vi "Scope_5782_6channel.vi"() -> ()   [LabVIEW 2018]
uses:
  FPGA/DataMode.ctl
  <vilib>/Analysis/4window.llb/windowTd.ctl
  Host/Scope/controls/power_spectrum_unit.ctl
  Host/Scope5782/Scope/controls/5782_trigger_type.ctl
  Host/Scope/controls/Data_calc_mode.ctl
  Host/Scope/controls/Data_display_mode.ctl
  Host/Scope/controls/Graph_references.ctl
  Host/Scope/controls/graph_controls.ctl
  Host/Scope/controls/Channel_select_2fpga.ctl
  <vilib>/userdefined/High Color/nirio_resource_hc.ctl
  Host/Communication/Driver/RemoteConnection/RemoteReferences.ctl
  Host/FpgaRef/FpgaRef5761/ClockSource_5761.ctl
  Host/Scope/Scope5782_six_channel/Scope5782_six_channel.lvclass
  C:/PXIe/Workspace/Host/Scope/ScopeBase/ScopeBase.lvclass
  Host/Communication/Driver/RemoteConnection/RemoteConnection.lvclass
  Host/Scope/ScopeBase/ScopeBase.lvclass/ScopeBase.ctl
  FPGA/fpga_settings.ctl
  Host/Scope/Scope5782_six_channel/Scope5782_six_channel.lvclass/Scope5782_six_channel.ctl
  Host/Scope/controls/ScopeMode.ctl
  Host/FpgaRef/FpgaRef5761/FpgaRef5761.lvclass
  C:/PXIe/Workspace/Host/FpgaRef/FpgaRefBase/FpgaRefBase.lvclass
  Host/FpgaRef/FpgaRef5782/FpgaRef5782.lvclass
  Host/Communication/global_stop.vi
  <vilib>/FPGAPlugInAG/PXIe-7975R/niLvFpga_Open_PXIe-7975R.vi
  <vilib>/rvi/interface/common/dynamic/niFpgaDynamicAddResources.vi
  Host/Communication/response.ctl
  Host/Communication/driver_status.ctl
  <vilib>/rvi/interface/nirviOpenFPGA/nirviOpenFPGA.xnode
  FPGA Bitfiles/FPGAmain_5782_Fast_PID_X3R1Zvw8vDM.lvbitx
  FPGA Bitfiles/FPGAmain_5761_zuew0qNtRjU.lvbitx
  <vilib>/rvi/FXPMathLib/FxpInterpret/XNode/nifxpmath_Interpret.xnode
  Host/Communication/Driver/TcpServerDriver/TcpServerDriver.lvclass
  Host/Scope/ScopeBase/ScopeBase.lvclass
  Host/FpgaRef/FpgaRefBase/FpgaRefBase.lvclass
  <vilib>/Analysis/NI_AALPro.lvlib
panel:
  in  "Tab Control":T1(tab)
  in  "Fequency [kHz]":dbl format="%#_8g"
  in  "a":fxp<+/-,16,2>
  in  "b":fxp<+/-,16,2>
  in  "Feedback":bool
  in  "Ki*T":fxp<+/-,32,4>
  in  "Kd/T":fxp<+/-,32,4>
  in  "Kp":fxp<+/-,32,4>
  in  "Feedback AM":bool caption="Feedback"
  in  "Ki*T AM":fxp<+/-,32,4> caption="Ki*T"
  in  "Kd/T AM":fxp<+/-,32,4> caption="Kd/T"
  in  "Kp AM":fxp<+/-,32,4> caption="Kp"
  in  "Feedback delay":u32
  in  "Trigger delay":u32
  in  "Acquire samples":u32
  in  "ch2 DC offset":dbl caption="DC offset\nChannel 2"
  in  "ch3 DC offset":dbl caption="DC offset\nChannel 3"
  in  "ch0 DC offset 2":dbl caption="DC offset\nChannel 0"
  in  "ch1 DC offset 2":dbl caption="DC offset\nChannel 1"
  in  "ch0 DC offset":dbl caption="DC offset\nChannel 0"
  in  "ch1 DC offset":dbl caption="DC offset\nChannel 1"
  in  "Setpoint":path
  in  "Beam":path
  in  "Feed forward":path
  in  "show setpoint":bool
  in  "show beam":bool
  in  "show feedforward":bool
  in  "Setpoint enabled":bool
  in  "Beam/FF enabled":bool
  in  "Cavity model":bool
  in  "w12":dbl format="%#_12g"
  in  "R1":dbl
  in  "w1":dbl
  in  "Q1":dbl
  in  "K1":dbl
  in  "S":dbl=0.001 min=0.001 max=1000.0 format="%#_12g"
  in  "Input delay 5761":u32
  in  "Input delay 5782":u32
  in  "5761 resource":T2="PXI2Slot11"
  in  "5782 resource":T2="PXI2Slot18"
  in  "High speed transfer to host":bool=TRUE
  in  "Output enabled":bool=TRUE
  in  "Output delay delta":dbl(slide) scale=0.0..6.0
  in  "Output delay":dbl(slide) scale=0.0..6.0
  in  "Output mixer fequency [MHz]":dbl
  in  "Trigger":T3
  in  "Mode":T4
  in  "Mixer freq [MHz]":dbl
  in  "unwrap phase":bool
  in  "#bins":i32=1 min=1 max=16
  in  "Unit":T5
  in  "Window":T6=1 items=["Rectangle"=0, "Hanning"=1, "Hamming"=2, "Blackman-Harris"=3, "Exact Blackman"=4, "Blackman"=5, "Flat Top"=6, "4 Term B-Harris "=7, "7 Term B-Harris"=8, "Low Sidelobe"=9, "Blackman Nuttall"=11, "Triangle"=30, "Bartlett-Hanning"=31, "Bohman"=32, "Parzen"=33, "Welch"=34, "Kaiser"=60, "Dolph-Chebyshev"=61, "Gaussian"=62]
  in  "Chart length":i32=400000
  in  "Trigmode":enum32{"Triggered", "Continuous"}(radio)
  in  "Reference for phase":T7
  in  "Graph_refs":T8
  out "Lower chart":dbl[][](graph)
  out "Upper chart":dbl[][](graph)
  out "Lower graph":i16[][](graph)
  in  "Buffer":T10
  in  "Display":T11
  out "stop 2":bool
  in  "Zoom freq X":bool
  in  "Zoom freq Y":bool
  in  "Zoom time Y":bool
  in  "Zoom time X":bool
  in  "Samples per 5782 record":i32
  in  "Phase offset (deg)":dbl
  in  "Fequency [MHz]":dbl format="%#_8g"
  out "freqdata":cluster{"f0":dbl, "df":dbl, "magnitude":dbl[]}[](graph)
  out "Upper graph":i16[][](graph)
  in  "Rumode":bool
  in  "Singleshot":bool
  out "error IO":errorcluster
  in  "stop":bool
  # "FPGA setup"
  # "ns"
  # "Output delay"
  # "ps"
  # "Output delay delta"
  # "Auto Zoom"
  # "FFT"
  # "Auto Zoom"
  # "Amplitude modulation"
  # "Phase"
  # "Amplitude"
  # "Delays"
  # "5782"
  # "V"
  # "V"
  # "5761"
  # "V"
  # "V"
  # "V"
  # "V"
  # "Simulated data"
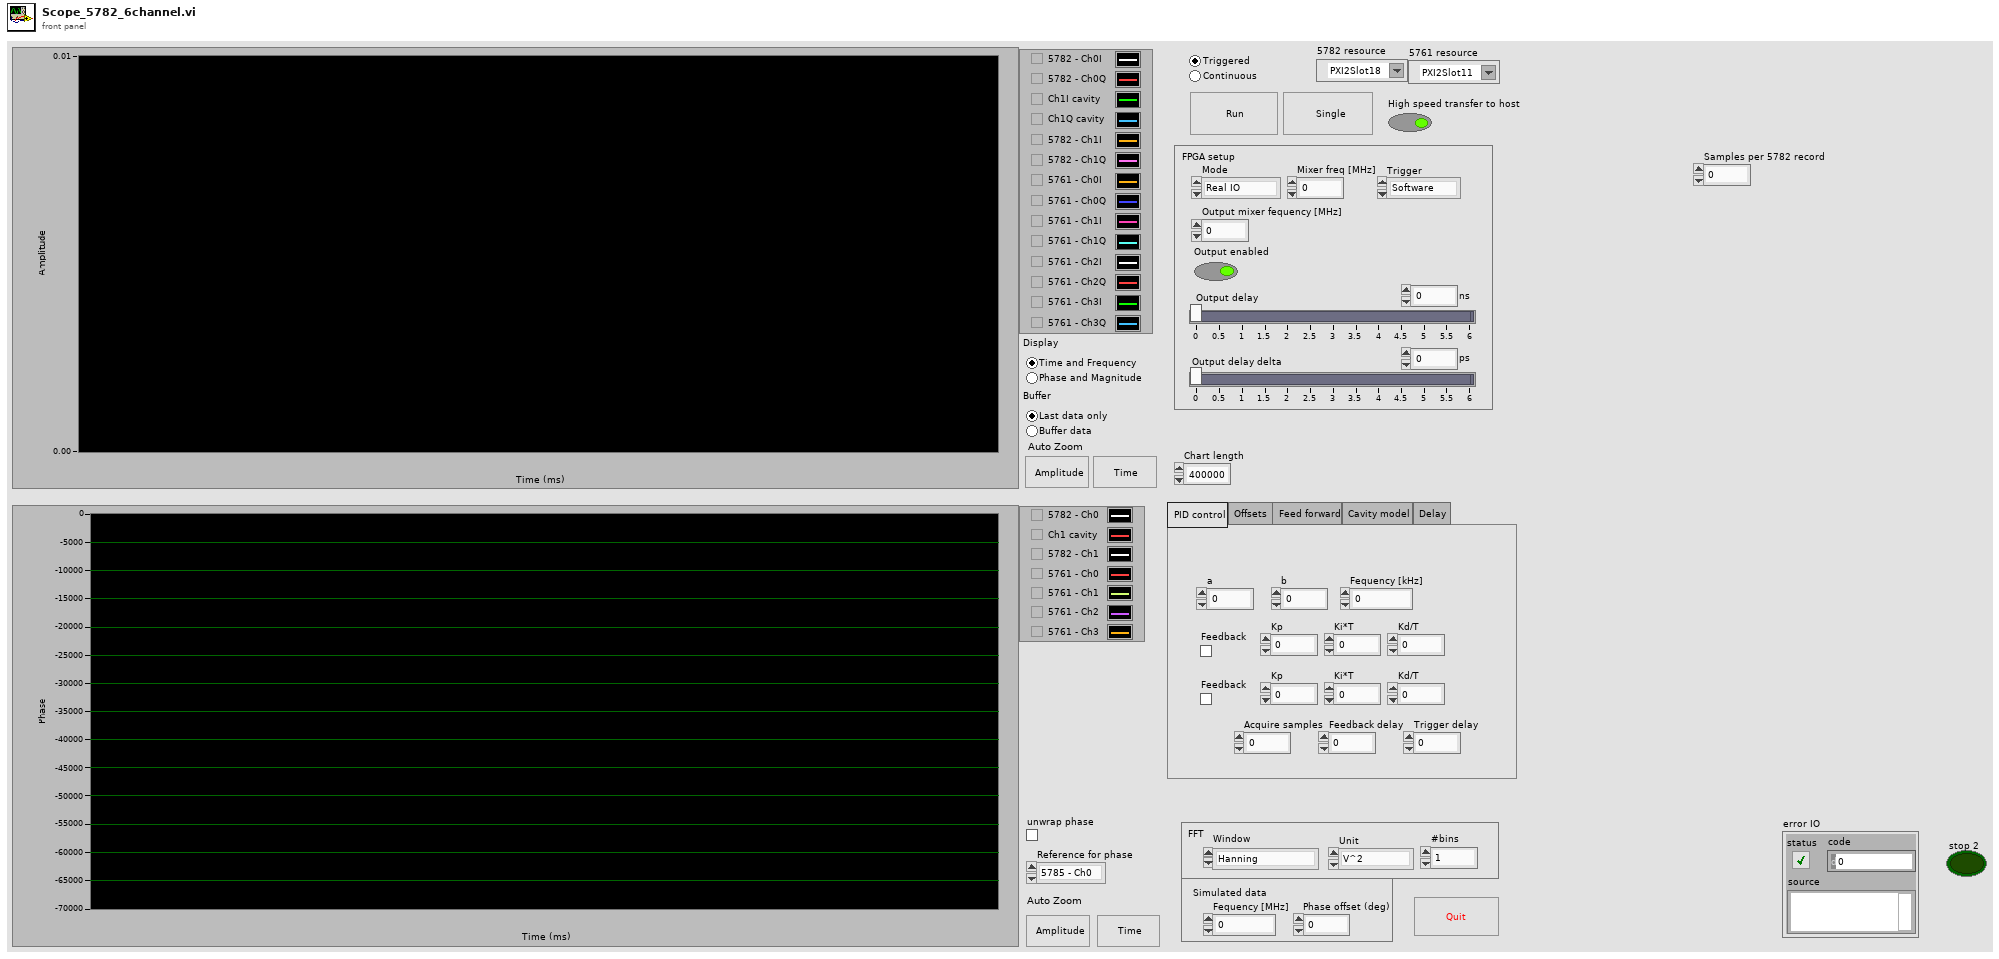
[diagram p1: front panel]
types:
  T1 = enum32{"PID control", "Offsets", "Feed forward", "Cavity model", "Delay"}
  T2 = typedef "nirio_resource_hc.ctl" = tag
  T3 = typedef "5782_trigger_type.ctl" = enum16{"Software", "Trigger input"}
  T4 = typedef "DataMode.ctl" = enum16{"Real IO", "Simulated"}
  T5 = typedef "power_spectrum_unit.ctl" = enum16{"V^2", "V", "dBV"}
  T6 = typedef "NI_AALPro.lvlib/windowTd.ctl" = u32
  T7 = typedef "Channel_select_2fpga.ctl" = enum16{"5785 - Ch0", "5785 - Ch1 cavity", "5785 - Ch1", "5761 - Ch0", "5761 - Ch1", "5761 - Ch2", "5761 - Ch3"}
  T8 = typedef "Graph_references.ctl" = cluster{"upper":T9, "lower":T9, "Freq graph":refnum<vi>}
  T9 = typedef "graph_controls.ctl" = cluster{"Graph":refnum<vi>, "Time btn":refnum<vi>, "Amplitude btn":refnum<vi>, "Chart":refnum<vi>}
  T10 = typedef "Data_display_mode.ctl" = enum32{"Last data only", "Buffer data"}
  T11 = typedef "Data_calc_mode.ctl" = enum32{"Time and Frequency", "Phase and Magnitude"}
  T12 = enum8{"Internal Clock PLL Off", "Internal Clock PLL On (REF IN)", "External Clock (CLK_IN)", "Internal Clock PLL On (IoModSyncClk)"}
  T13 = typedef "ClockSource_5761.ctl" = enum8{"Internal Clock PLL Off", "Internal Clock PLL On (CLK_IN)", "External Clock (CLK_IN)", "Internal Clock PLL On (IoModSyncClk)", "External Clock (IoModSyncClk)"}
  T14 = typedef "RemoteConnection.lvclass/RemoteReferences.ctl" = cluster{"a":refnum<vi>, "b":refnum<vi>, "fm":refnum<vi>, "Output delay":refnum<vi>, "Output delay delta":refnum<vi>}
  T15 = typedef "response.ctl" = cluster{"driver status":T16, "Sender":string, "Type":i32, "Variant":variant}
  T16 = typedef "driver_status.ctl" = enum16{"Normal", "Startup", "Connection lost", "Reconnected", "Timeout", "Idle", "Busy"}
  T17 = typedef "message_queue.ctl" = refnum<queue>
  T18 = typedef "fpga_settings.ctl" = enum16{"Feedback Enable", "New FIR coeffs", "FIR shift", "Enable filter", "Set Downsample", "Downsample", "CIC Gain", "Record length", "Trigger samples", "Quiet time", "a_am", "b_am", "Use fixed delay", "fixed sin_fi", "fixed cos_fi", "Ki*Tau", "Kp", "Kd_Tau", "Fi_start", "Fi_delta", "DC_offs 0", "DC_offs 1", "DC_offs 2", "DC_offs 3", "Ki*Tau am", "Kp am", "Kd_Tau am", "Feedback AM", "Trigger delay", "Feedback delay", "Setpoint enable", "Beam enable", "Samples to acquire", "Cavity Enable", "Cavity C1", "Cavity C2", "Cavity C3", "Cavity C4", "Cavity C5", "Input delay"}
  T19 = typedef "ScopeMode.ctl" = enum16{"Stopped", "Single", "Running", "Continuous"}
  T20 = typedef "Feedforward.ctl" = cluster{"Beam I":dbl[], "Beam Q":dbl[], "Feedforward I":dbl[], "Feedforward Q":dbl[], "Setpoint I":dbl[], "Setpoint Q":dbl[]}
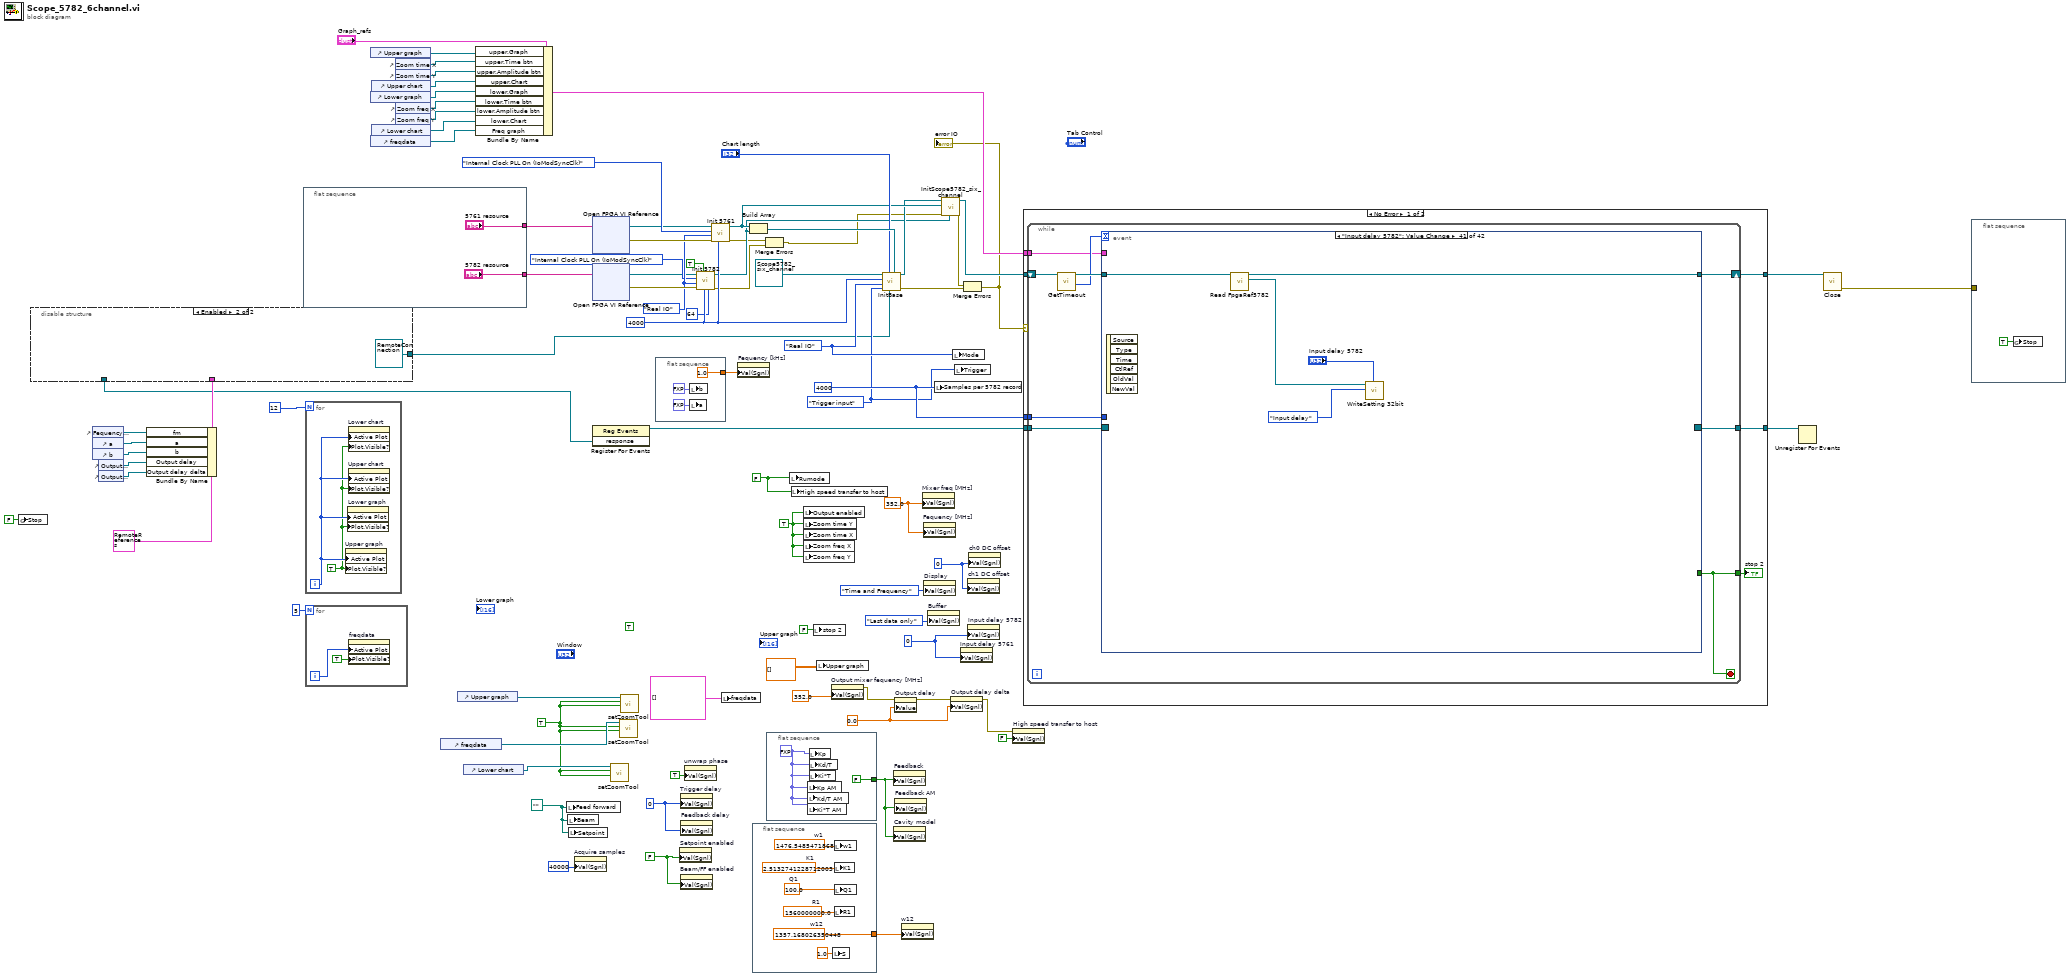
[diagram p0: block diagram]
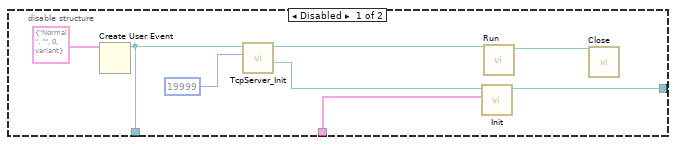
[diagram p2: hidden frame]
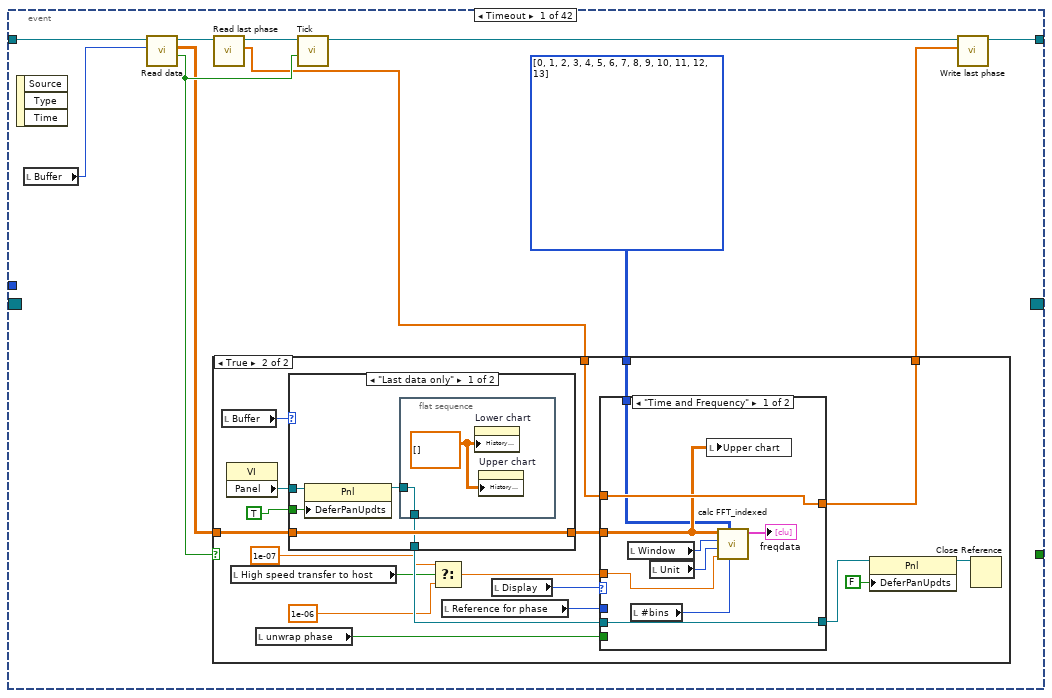
[diagram p3: hidden frame]
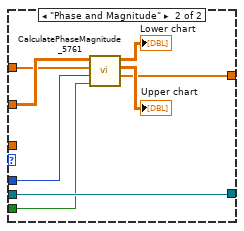
[diagram p6: hidden frame]
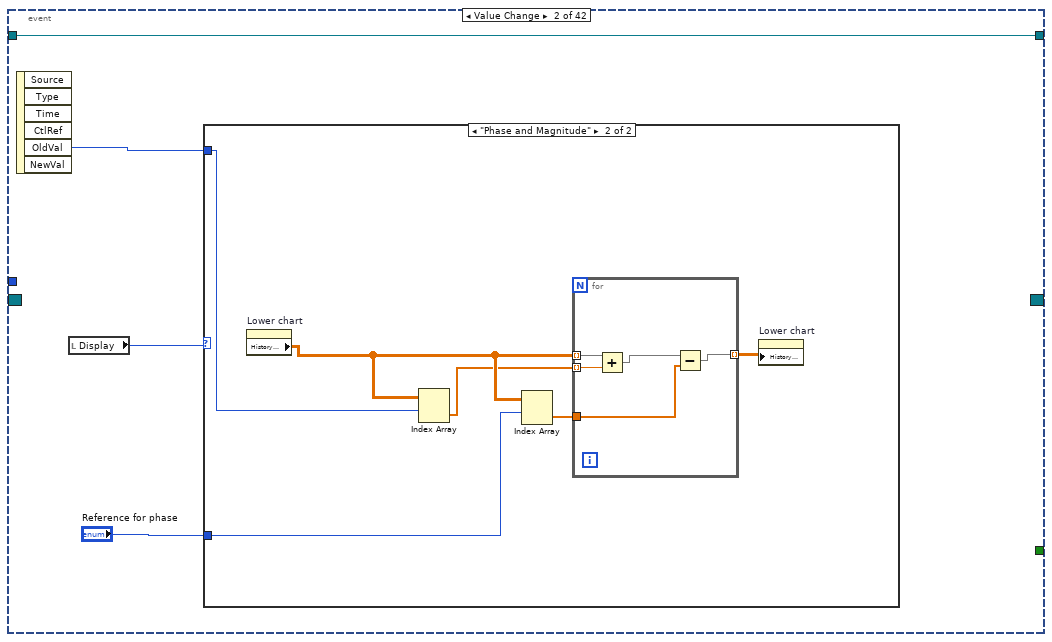
[diagram p7: hidden frame]
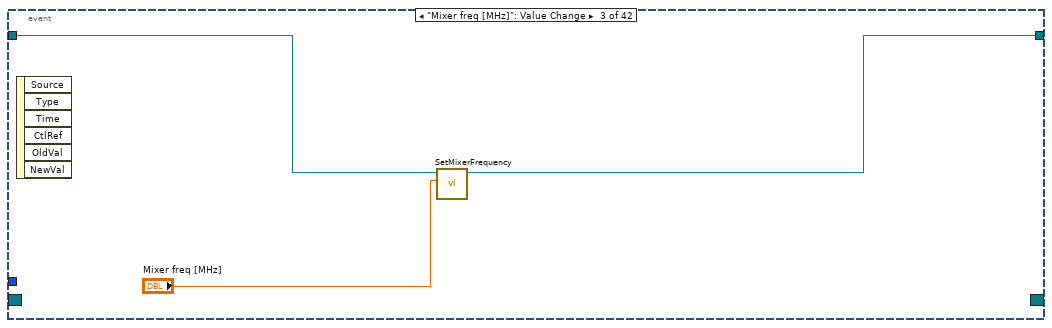
[diagram p9: hidden frame]
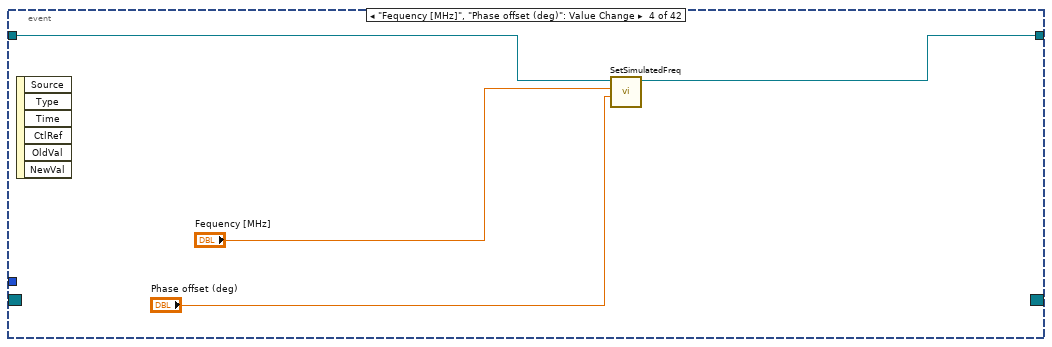
[diagram p10: hidden frame]
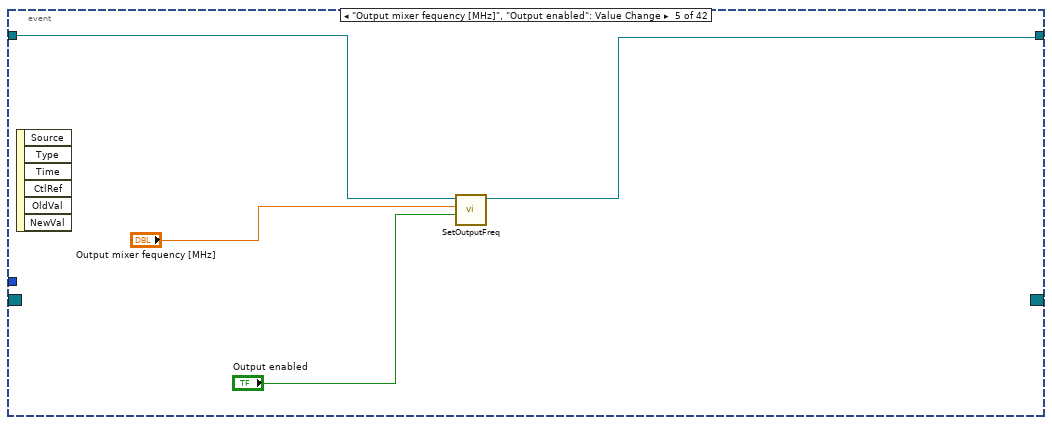
[diagram p11: hidden frame]
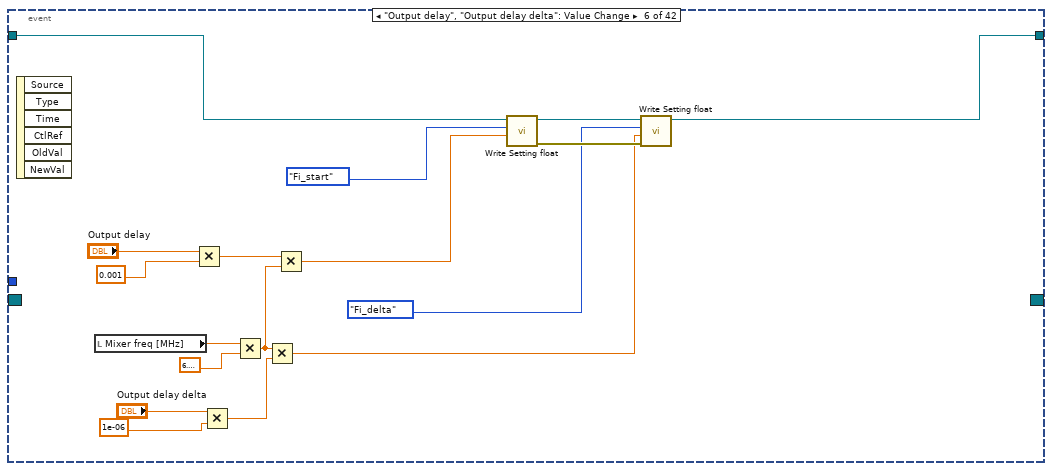
[diagram p12: hidden frame]
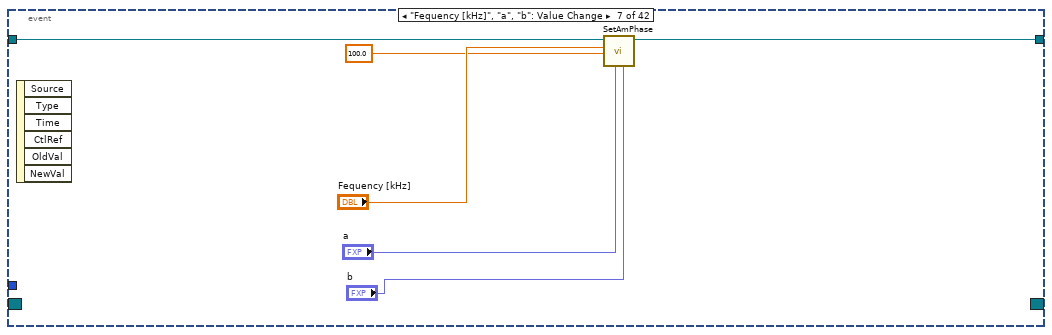
[diagram p13: hidden frame]
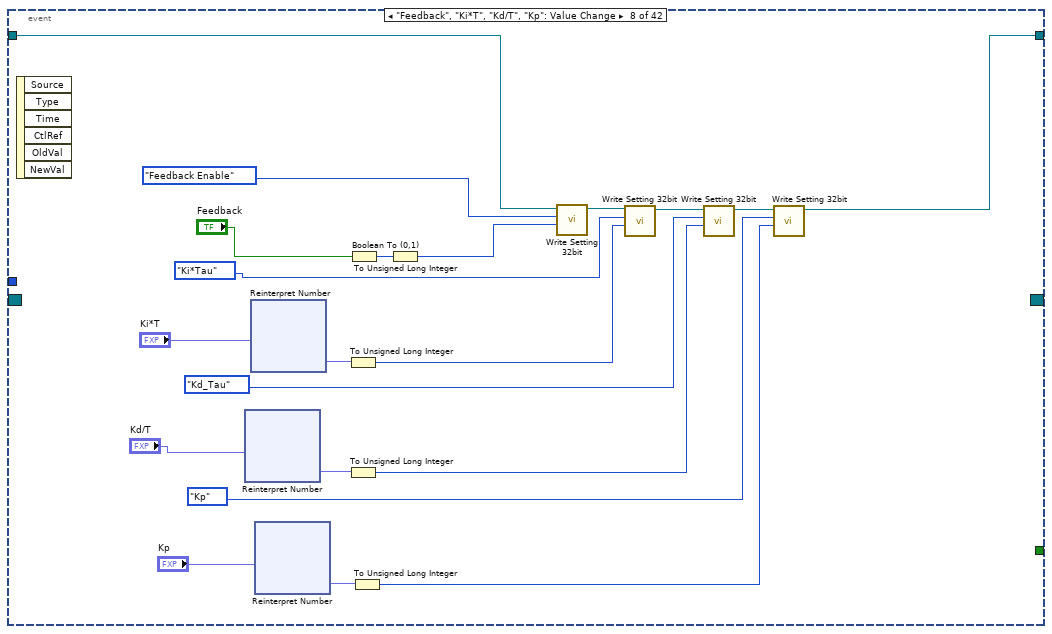
[diagram p14: hidden frame]
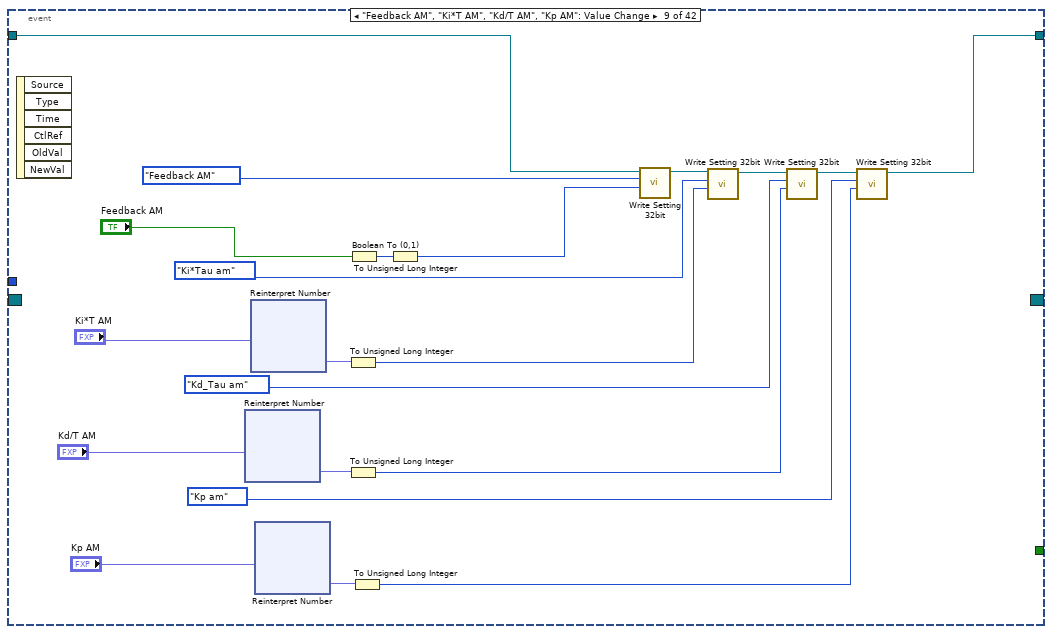
[diagram p15: hidden frame]
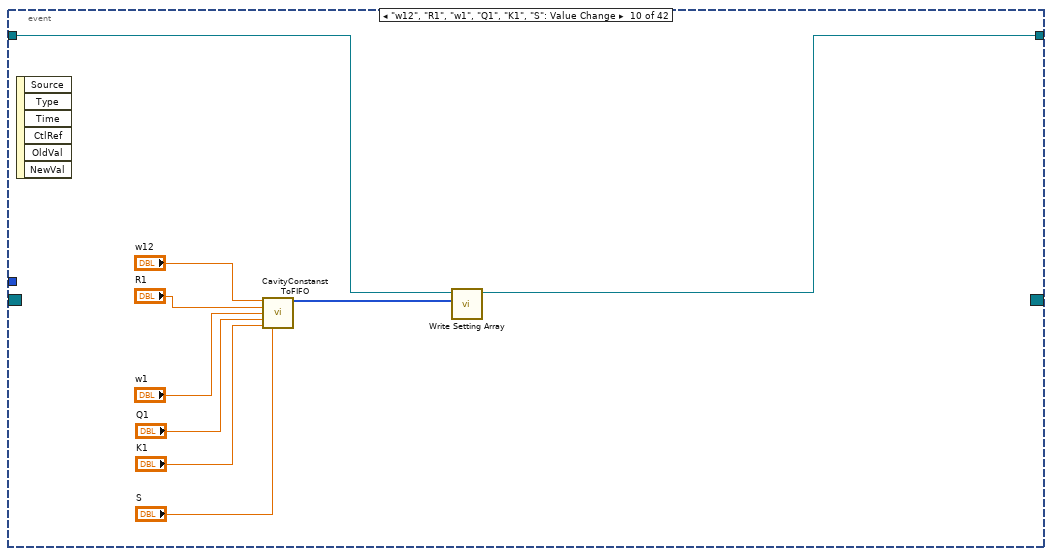
[diagram p16: hidden frame]
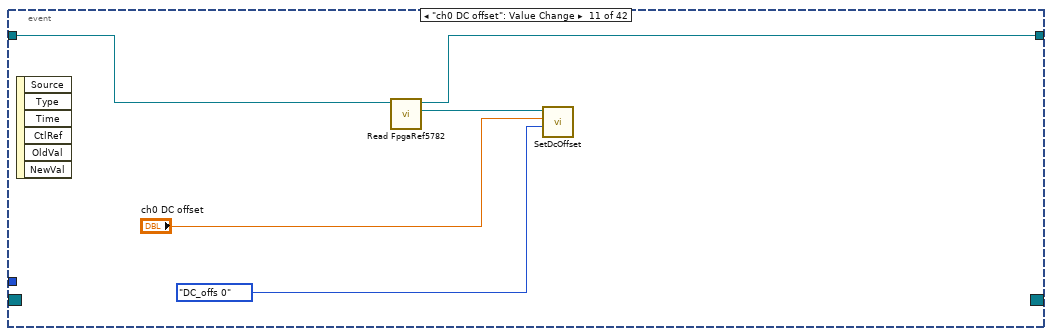
[diagram p17: hidden frame]
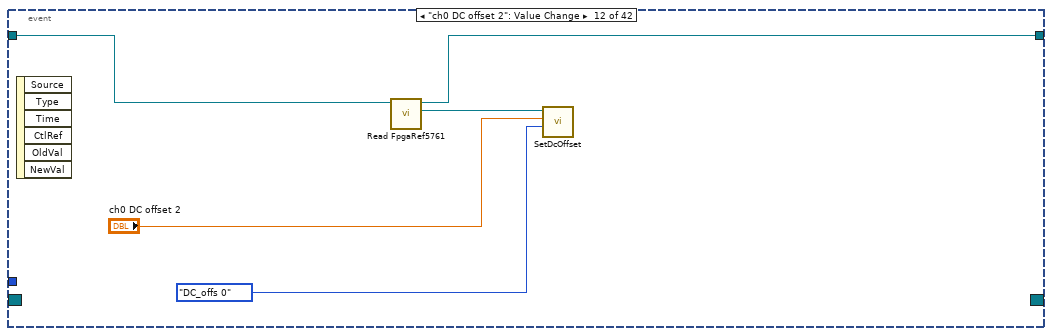
[diagram p18: hidden frame]
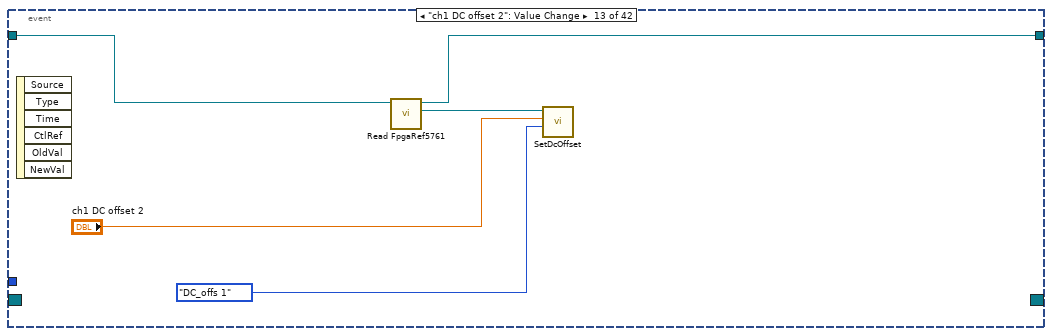
[diagram p19: hidden frame]
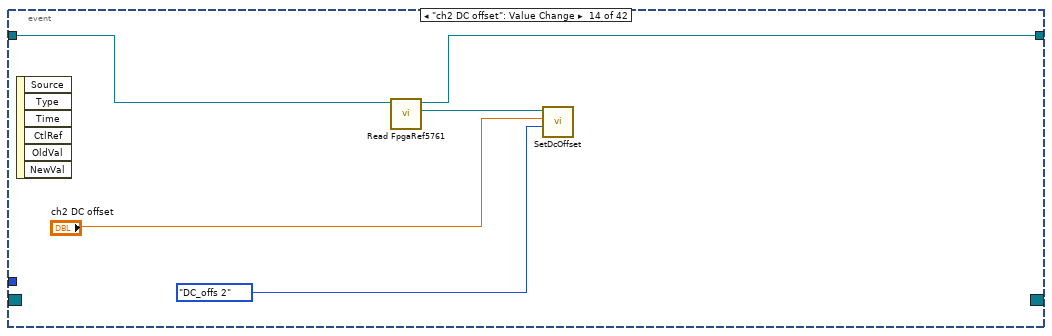
[diagram p20: hidden frame]
diagram:
  w1 = u32 0 ("Value (Signaling)")
  w18 = u16 4000 ("Samples to aqcuire")
  w14 = DataMode."Real IO" ("Mode")
  w27 = DataMode."Real IO" ("Mode")
  w35 = path "" ("Feed forward")
  w36 = FALSE ("Value (Signaling)")
  w37 = u32 0 ("Value (Signaling)")
  w56 = i16 0 ("Value (Signaling)")
  w57 = 0.0 ("Value (Signaling)")
  w26 = 5782_trigger_type."Trigger input" ("Trigger")
  w46 = TRUE ("Zoom  X")
  w42 = TRUE ("Rumode")
  w41 = 4000 ("Samples to aqcuire")
  (unwired) TRUE ("Rumode")
  w40 = FALSE ("Rumode")
  w81 = 352.0 ("Mixer requency [MHz]")
  n1 = global write "global_stop.vi" "Stop"(FALSE ("Stop")) -> ()
  n2 = control-ref of="Fequency [kHz]"() -> (w50:refnum<vi>)
  n3 = control-ref of="a"() -> (w51:refnum<vi>)
  n4 = control-ref of="b"() -> (w49:refnum<vi>)
  n5 = control-ref of="Output delay"() -> (w45:refnum<vi>)
  n6 = control-ref of="Output delay delta"() -> (w44:refnum<vi>)
  n7 = Bundle By Name(cluster=T14 {"a"=refnum, "b"=refnum, "fm"=refnum, "Output delay"=refnum, "Output delay delta"=refnum} ("refs"), "fm"=w50, "a"=w51, "b"=w49, "Output delay"=w45, "Output delay delta"=w44) -> (w54:T14)
  n8 = disable-structure shown="Enabled" {
    disable-tunnel: w54 -> [w91 _]
    disable-tunnel: [w86 _] -> w48
    disable-tunnel: [w84 refnum<class "RemoteConnection.lvclass"> refnum ("RemoteConnection")] -> w25
    frame Disabled {
      n9 = Create User Event(user event datatype=T15 {"driver status"=enum."Normal", "Sender"="", "Type"=0, "Variant"=variant} ("response")) -> (user event=w86:refnum<user-event>)  [unwired: 1 in, 1 out]
      n10 = call "TcpServer_Init.vi"("local port"=u16 19999, "response event"=w86) -> ("Message queue"=w90:T17, "TcpServerDriver"=w88:refnum<class "TcpServerDriver.lvclass">)  [unwired: 8 in]
      n11 = call "Init.vi"("refs"=w91, "server queue"=w90) -> ("RemoteConnection"=w84:refnum<class "RemoteConnection.lvclass">)  [unwired: 9 in]
      n12 = call-dynamic "Run.vi"("BaseDriver in"=w88) -> ("BaseDriver out"=w89:refnum<class "TcpServerDriver.lvclass">)  [unwired: 9 in, 1 out]
      n13 = call-dynamic "Close.vi"("BaseDriver in"=w89) -> ()  [unwired: 9 in, 2 out]
    }
    frame Enabled {
    }
  }
  n14 = flat-sequence {
    tunnel: ["5761 resource"] -> w29
    tunnel: ["5782 resource"] -> w28
    frame #0 {
    }
  }
  n15 = for {
    N: 12 -> [_]
    i -> [w96]
    w95 = TRUE ("Plot.Visible")
    n16 = property on="Upper graph" class="WFGraph (strict)"("Active Plot"=w96, "Plot.Visible?"=w95) -> ()  [unwired: 2 in, 2 out]
    n17 = property on="Lower graph" class="WFGraph (strict)"("Active Plot"=w96, "Plot.Visible?"=w95) -> ()  [unwired: 2 in, 2 out]
    n18 = property on="Lower chart" class="WFChart (strict)"("Active Plot"=w96, "Plot.Visible?"=w95) -> ()  [unwired: 2 in, 2 out]
    n19 = property on="Upper chart" class="WFChart (strict)"("Active Plot"=w96, "Plot.Visible?"=w95) -> ()  [unwired: 2 in, 2 out]
  }
  n20 = for {
    N: 5 -> [_]
    i -> [w97]
    n21 = property on="freqdata" class="WFGraph (strict)"("Active Plot"=w97, "Plot.Visible?"=TRUE ("Plot.Visible")) -> ()  [unwired: 2 in, 2 out]
  }
  n22 = control-ref of="Upper graph"() -> (w71:refnum<vi>)
  n23 = control-ref of="Lower graph"() -> (w67:refnum<vi>)
  n24 = control-ref of="freqdata"() -> (w63:refnum<vi>)
  n25 = control-ref of="Upper chart"() -> (w68:refnum<vi>)
  n26 = control-ref of="Lower chart"() -> (w64:refnum<vi>)
  n27 = control-ref of="Zoom time X"() -> (w70:refnum<vi>)
  n28 = control-ref of="Zoom time Y"() -> (w69:refnum<vi>)
  n29 = control-ref of="Zoom freq X"() -> (w66:refnum<vi>)
  n30 = control-ref of="Zoom freq Y"() -> (w65:refnum<vi>)
  n31 = control-ref of="freqdata"() -> (w74:refnum<vi>)
  n32 = control-ref of="Upper graph"() -> (w75:refnum<vi>)
  n33 = control-ref of="Lower chart"() -> (w47:refnum<vi>)
  n34 = Bundle By Name(cluster="Graph_refs", "upper.Graph"=w71, "upper.Time btn"=w70, "upper.Amplitude btn"=w69, "upper.Chart"=w68, "lower.Graph"=w67, "lower.Time btn"=w66, "lower.Amplitude btn"=w65, "lower.Chart"=w64, "Freq graph"=w63) -> (w62:T8)
  n35 = local write "Feed forward"(w35) -> ()
  n36 = local write "Beam"(w35) -> ()
  n37 = local write "Setpoint"(w35) -> ()
  n38 = property on="Acquire samples" class="DigNum (strict)"("Val(Sgnl)"=u32 40000 ("Value (Signaling)")) -> ()  [unwired: 2 in, 2 out]
  n39 = register-events(w48) -> (reference out=w78:refnum<event-registration>)  [unwired: 2 in, 1 out]
  n40 = xnode "Open FPGA VI Reference"("resource name"=w29) -> ("FPGA VI Reference Out"=w2:refnum<k20>, "error out"=w16:errorcluster)  [unwired: 1 in]
  n41 = xnode "Open FPGA VI Reference"("resource name"=w28) -> ("FPGA VI Reference Out"=w3:refnum<k20>, "error out"=w17:errorcluster)  [unwired: 1 in]
  n42 = call "setZoomTool.vi"("Zoom Y"=w46, "Zoom  X"=w46, "reference"=w47) -> ()  [unwired: 9 in]
  n43 = call "setZoomTool.vi"("Zoom Y"=w46, "Zoom  X"=w46, "reference"=w74) -> ()  [unwired: 9 in]
  n44 = call "setZoomTool.vi"("Zoom Y"=w46, "Zoom  X"=w46, "reference"=w75) -> ()  [unwired: 9 in]
  n45 = flat-sequence {
    tunnel: [1.0 ("Value (Signaling)")] -> w55
    frame #0 {
      n46 = local write "b"(fxp<+/-,16,2> 0.0 ("b")) -> ()
      n47 = local write "a"(fxp<+/-,16,2> 1.0 ("a")) -> ()
    }
  }
  n48 = property on="Setpoint enabled" class="Bool (strict)"("Val(Sgnl)"=w36) -> ()  [unwired: 2 in, 2 out]
  n49 = property on="Trigger delay" class="DigNum (strict)"("Val(Sgnl)"=w37) -> ()  [unwired: 2 in, 2 out]
  n50 = property on="Beam/FF enabled" class="Bool (strict)"("Val(Sgnl)"=w36) -> ()  [unwired: 2 in, 2 out]
  n51 = property on="Feedback delay" class="DigNum (strict)"("Val(Sgnl)"=w37) -> ()  [unwired: 2 in, 2 out]
  n52 = property on="unwrap phase" class="Bool (strict)"("Val(Sgnl)"=TRUE ("Value (Signaling)")) -> ()  [unwired: 2 in, 2 out]
  n53 = call "Init 5782.vi"("User Data 1"=u8 64, "Record length"=w18, "Use 1Mhz clock"=TRUE, "error in (no error)"=w17, "Mode"=w14, "Clock Source"=T12."Internal Clock PLL On (IoModSyncClk)", "FPGA ref"=w3) -> ("error out"=w8:errorcluster, "FpgaRef5782 Out"=w11:refnum<class "FpgaRef5782.lvclass">)  [unwired: 3 in]
  n54 = call "Init 5761.vi"("Record length"=w18, "error in (no error)"=w16, "Mode"=w14, "Clock Source"=ClockSource_5761."Internal Clock PLL On (IoModSyncClk)", "FPGA ref"=w2) -> ("error out"=w9:errorcluster, "FpgaRef5761 out"=w21:refnum<class "FpgaRef5761.lvclass">)  [unwired: 5 in]
  n55 = local write "freqdata"(cluster{"f0":dbl, "df":dbl, "magnitude":dbl[]}[] [] ("freqdata")) -> ()
  n56 = property on="Fequency [kHz]" class="DigNum (strict)"("Val(Sgnl)"=w55) -> ()  [unwired: 2 in, 2 out]
  n57 = Build Array(w21, w11) -> (w30:refnum<class "FpgaRefBase.lvclass">[])
  n58 = flat-sequence {
    tunnel: [w103] -> w32
    frame #0 {
      w104 = 2.5132741228712003  # K1
      w105 = 100.0  # Q1
      w106 = 1476.54854718683  # w1
      w107 = 1560000000.0  # R1
      w103 = 1357.168026350448  # w12
      n59 = local write "S"(1.0 ("S")) -> ()
      n60 = local write "w1"(w106) -> ()
      n61 = local write "K1"(w104) -> ()
      n62 = local write "Q1"(w105) -> ()
      n63 = local write "R1"(w107) -> ()
    }
  }
  n64 = Merge Errors(w9, w8) -> (w7:errorcluster)
  n65 = flat-sequence {
    tunnel: [FALSE] -> w33
    frame #0 {
      w108 = fxp<+/-,32,4> 0.0 ("Kp")
      n66 = local write "Kp AM"(w108) -> ()
      n67 = local write "Kd/T AM"(w108) -> ()
      n68 = local write "Ki*T AM"(w108) -> ()
      n69 = local write "Kp"(w108) -> ()
      n70 = local write "Kd/T"(w108) -> ()
      n71 = local write "Ki*T"(w108) -> ()
    }
  }
  n72 = local write "Rumode"(w40) -> ()
  n73 = local write "High speed transfer to host"(w40) -> ()
  n74 = local write "Output enabled"(w42) -> ()
  n75 = local write "Zoom time Y"(w42) -> ()
  n76 = local write "Zoom time X"(w42) -> ()
  n77 = local write "Zoom freq X"(w42) -> ()
  n78 = local write "Zoom freq Y"(w42) -> ()
  n79 = local write "stop 2"(FALSE ("stop 2")) -> ()
  n80 = local write "Upper graph"(dbl[][] [] ("Timedata")) -> ()
  n81 = property on="Output mixer fequency [MHz]" class="DigNum (strict)"("Val(Sgnl)"=352.0 ("Mixer requency [MHz]")) -> (error out=w58:errorcluster)  [unwired: 2 in, 1 out]
  n82 = call "InitBase.vi"("FPGA refs"=w30, "RemoteConnection"=w25, "Chart length"="Chart length", "Trigger"=w26, "data mode"=w27, "Samples Per Trigger"=w18, "ScopeBase in"=refnum<class "Scope5782_six_channel.lvclass"> refnum) -> ("error out"=w5:errorcluster, "ScopeBase out"=w20:refnum<class "Scope5782_six_channel.lvclass">)  [unwired: 3 in]
  n83 = property on="Feedback" class="Bool (strict)"("Val(Sgnl)"=w33) -> ()  [unwired: 2 in, 2 out]
  n84 = property on="Cavity model" class="Bool (strict)"("Val(Sgnl)"=w33) -> ()  [unwired: 2 in, 2 out]
  n85 = property on="Output delay" class="Slide (strict)"(error in=w58, "Value"=w57) -> (error out=w59:errorcluster)  [unwired: 1 in, 1 out]
  n86 = property on="Feedback AM" class="Bool (strict)"("Val(Sgnl)"=w33) -> ()  [unwired: 2 in, 2 out]
  n87 = property on="w12" class="DigNum (strict)"("Val(Sgnl)"=w32) -> ()  [unwired: 2 in, 2 out]
  n88 = property on="Mixer freq [MHz]" class="DigNum (strict)"("Val(Sgnl)"=w81) -> ()  [unwired: 2 in, 2 out]
  n89 = property on="Fequency [MHz]" class="DigNum (strict)"("Val(Sgnl)"=w81) -> ()  [unwired: 2 in, 2 out]
  n90 = property on="Display" class="RadioBtnsControl (strict)"("Val(Sgnl)"=Data_calc_mode."Time and Frequency" ("Value (Signaling)")) -> ()  [unwired: 2 in, 2 out]
  n91 = property on="Buffer" class="RadioBtnsControl (strict)"("Val(Sgnl)"=enum32{"Last data only", "Buffer data"}."Last data only" ("Value (Signaling)")) -> ()  [unwired: 2 in, 2 out]
  n92 = local write "Samples per 5782 record"(w41) -> ()
  n93 = call "InitScope5782_six_channel.vi"("FpgaRef5782"=w11, "error in (no error)"=w7, "FpgaRef5761"=w21, "Scope5785_six_channel"=w20) -> ("error out"=w6:errorcluster, "Scope5785_six_channel out"=w19:refnum<class "Scope5782_six_channel.lvclass">)  [unwired: 6 in]
  n94 = property on="Output delay delta" class="Slide (strict)"(error in=w59, "Val(Sgnl)"=w57) -> (error out=w39:errorcluster)  [unwired: 1 in, 1 out]
  n95 = local write "Mode"(w27) -> ()
  n96 = local write "Trigger"(w26) -> ()
  n97 = property on="Input delay 5761" class="DigNum (strict)"("Val(Sgnl)"=w1) -> ()  [unwired: 2 in, 2 out]
  n98 = Merge Errors(w6, w5) -> (w4:errorcluster)
  "error IO" <- w4
  n99 = property on="ch1 DC offset" class="DigNum (strict)"("Val(Sgnl)"=w56) -> ()  [unwired: 2 in, 2 out]
  n100 = property on="Input delay 5782" class="DigNum (strict)"("Val(Sgnl)"=w1) -> ()  [unwired: 2 in, 2 out]
  n101 = property on="ch0 DC offset" class="DigNum (strict)"("Val(Sgnl)"=w56) -> ()  [unwired: 2 in, 2 out]
  n102 = property on="High speed transfer to host" class="Bool (strict)"(error in=w39, "Val(Sgnl)"=FALSE ("Value (Signaling)")) -> ()  [unwired: 1 in, 2 out]
  n103 = case shown="No Error" w4 {
    tunnel: w19 -> [w116 w498]
    tunnel: [w115 w498] -> w23
    tunnel: w78 -> [w114 w497]
    tunnel: [w113 w497] -> w77
    tunnel: w62 -> [w111 _]
    tunnel: w41 -> [w110 _]
    frame No Error {
      n104 = while {
        shift-right: [w117] -> w115
        shift-left: w116 -> [w125]
        tunnel: w114 -> [w122]
        tunnel: [w121] -> w113
        tunnel: [w120] -> w112
        tunnel: w111 -> [w119]
        tunnel: w110 -> [w118]
        stop <- w120 stop-if-true
        n105 = call "GetTimeout.vi"("ScopeBase in"=w125) -> ("Time left"=w123:i32, "ScopeBase out"=w124:refnum<class "Scope5782_six_channel.lvclass">)  [unwired: 8 in, 1 out]
        n106 = event shown="[40] \"Input delay 5782\": Value Change" {
          selector: w122 -> [_ _ _ _ _ _ _ _ _ _ _ _ _ _ _ _ _ _ _ _ _ _ _ _ _ _ _ _ _ _ _ _ _ _ _ _ _ _ _ _ _ _]
          dyn-events: [_ _ _ _ _ _ _ _ _ _ _ _ _ _ _ _ _ _ _ _ _ _ _ _ _ _ _ _ _ _ _ _ _ _ _ _ _ _ _ _ _ _] -> w121
          timeout: w123 -> [_ _ _ _ _ _ _ _ _ _ _ _ _ _ _ _ _ _ _ _ _ _ _ _ _ _ _ _ _ _ _ _ _ _ _ _ _ _ _ _ _ _]
          tunnel: [_ _ _ _ _ _ _ _ _ _ _ _ _ _ _ _ _ _ _ _ _ _ _ _ _ _ _ _ _ _ _ "stop" _ _ _ _ _ _ _ _ _ _] -> w120
          tunnel: w124 -> [w136 w186 w200 w202 w208 w216 w231 w244 w262 w275 w286 w291 w296 w301 w306 w314 w317 w321 w334 w345 w360 w361 w370 w380 w387 w391 w396 w413 w414 w419 w428 w429 w436 w447 w452 w458 w465 w470 w475 w482 w491 w496]
          tunnel: [w129 w186 w198 w201 w205 w209 w230 w240 w261 w274 w285 w290 w295 w300 w305 w308 w316 w322 w333 w346 w359 w362 w369 w379 w385 w389 w392 w411 w415 w418 w428 w429 w436 w447 w452 w458 w465 w466 w474 w480 w487 w493] -> w117
          tunnel: w119 -> [_ _ _ _ _ _ _ _ _ _ _ _ _ _ _ _ _ _ _ _ _ _ _ _ _ _ _ _ _ _ _ _ _ _ _ _ w462 _ _ _ _ _]
          tunnel: w118 -> [_ _ _ _ _ _ _ _ _ _ _ _ _ _ _ _ _ _ _ _ _ _ _ _ _ _ w408 _ _ _ _ _ _ _ _ _ _ _ _ _ _ _]
          event Timeout {
            n107 = event-data() -> ()  [unwired: 1 in, 3 out]
            n108 = local read "Buffer"() -> (w135:T10)
            n109 = call-dynamic "Read data.vi"("Buffer mode"=w135, "Scope5785_six_channel"=w136) -> ("Any read?"=w132:bool, "Data"=w127:dbl[][], "Scope5785_six_channel out"=w134:refnum<class "Scope5782_six_channel.lvclass">)  [unwired: 6 in, 1 out]
            n110 = call "Read last phase.vi"("ScopeBase in"=w134) -> ("last phase"=w131:dbl[], "ScopeBase out"=w133:refnum<class "Scope5782_six_channel.lvclass">)  [unwired: 8 in, 1 out]
            n111 = case shown="True" w132 {
              tunnel: w127 -> [_ w153]
              tunnel: w131 -> [w137 w145]
              tunnel: [w137 w144] -> w128
              tunnel: i32[][] [[0, 1], [2, 3], [4, 5], [6, 7], [8, 9], [10, 11], [12, 13]] ("IQ indexes") -> [_ w138]
              frame False {
              }
              frame True {
                n112 = local read "Buffer"() -> (w155:T10)
                n113 = property class="VI"() -> ("Panel"=w148:refnum<vi>)  [unwired: 2 in, 2 out]
                n114 = local read "High speed transfer to host"() -> (w143:bool)
                n115 = local read "unwrap phase"() -> (w139:bool)
                n116 = case shown="\"Last data only\"" w155 {
                  tunnel: w153 -> [w161 w165]
                  tunnel: [w161 w165] -> w154
                  tunnel: w148 -> [w160 w164]
                  tunnel: TRUE ("Defer Panel Updates") -> [w158 _]
                  tunnel: [w157 w164] -> w146
                  frame "Last data only" {
                    n117 = property class="Pnl"(reference=w160, "DeferPanUpdts"=w158) -> (reference out=w159:refnum<vi>)  [unwired: 1 in, 1 out]
                    n118 = flat-sequence {
                      tunnel: w159 -> [w162]
                      tunnel: [w162] -> w157
                      frame #0 {
                        w163 = dbl[][] [] ("History Data")
                        n119 = property on="Lower chart" class="WFChart (strict)"("History Data"=w163) -> ()  [unwired: 2 in, 2 out]
                        n120 = property on="Upper chart" class="WFChart (strict)"("History Data"=w163) -> ()  [unwired: 2 in, 2 out]
                      }
                    }
                  }
                  frame "Buffer data" {
                  }
                }
                n121 = Select(t=1e-07 ("dt"), s=w143, f=1e-06 ("dt")) -> (s? t:f=w140:dbl)
                n122 = local read "Reference for phase"() -> (w152:T7)
                n123 = local read "Display"() -> (w156:T11)
                n124 = case shown="\"Time and Frequency\"" w156 {
                  tunnel: w154 -> [w167 w182]
                  tunnel: w152 -> [_ w179]
                  tunnel: [w171 w178] -> w150
                  tunnel: w146 -> [w171 w178]
                  tunnel: w145 -> [w169 w177]
                  tunnel: [w169 w176] -> w144
                  tunnel: w140 -> [w168 _]
                  tunnel: w139 -> [_ w175]
                  tunnel: w138 -> [w166 _]
                  frame "Time and Frequency" {
                    n125 = local read "Window"() -> (w172:T6)
                    n126 = local read "#bins"() -> (w170:i32)
                    n127 = local read "Unit"() -> (w173:T5)
                    n128 = local write "Upper chart"(w167) -> ()
                    n129 = call "calc FFT_indexed.vi"("#bins"=w170, "IQ indexes"=w166, "dt"=w168, "Unit"=w173, "Window"=w172, "data"=w167) -> ("Power Spectrum / PSD"=→"freqdata":cluster{"f0":dbl, "df":dbl, "magnitude":dbl[]}[])  [unwired: 5 in]
                  }
                  frame "Phase and Magnitude" {
                    n130 = call "CalculatePhaseMagnitude_5761.vi"("unwrap phase"=w175, "phase reference channel"=w179, "previous phase"=w177, "data"=w182) -> ("last phase"=w176:dbl[], "Magnitude"=→"Upper chart":dbl[][], "Phase"=→"Lower chart":dbl[][])  [unwired: 5 in]
                  }
                }
                n131 = property class="Pnl"(reference=w150, "DeferPanUpdts"=FALSE ("Defer Panel Updates")) -> (reference out=w149:refnum<vi>)  [unwired: 1 in, 1 out]
                n132 = Close Reference(reference=w149) -> ()  [unwired: 1 in, 1 out]
              }
            }
            n133 = call "Tick.vi"("Any elements read?"=w132, "ScopeBase in"=w133) -> ("ScopeBase out"=w130:refnum<class "Scope5782_six_channel.lvclass">)  [unwired: 8 in, 1 out]
            n134 = call "Write last phase.vi"("last phase"=w128, "ScopeBase in"=w130) -> ("ScopeBase out"=w129:refnum<class "Scope5782_six_channel.lvclass">)  [unwired: 8 in, 1 out]
          }
          event Value Change {
            n135 = event-data() -> ("OldVal"=w183:T7)  [unwired: 1 in, 5 out]
            n136 = local read "Display"() -> (w184:T11)
            n137 = case shown="\"Phase and Magnitude\"" w184 {
              tunnel: "Reference for phase" -> [_ w191]
              tunnel: w183 -> [_ w189]
              frame "Time and Frequency", Default {
              }
              frame "Phase and Magnitude" {
                n138 = property on="Lower chart" class="WFChart (strict)"() -> ("History Data"=w190:dbl[][])  [unwired: 2 in, 2 out]
                n139 = Index Array(array=w190, index (row)=w189) -> (element=w188:dbl[])  [unwired: 1 in]
                n140 = Index Array(array=w190, index (row)=w191) -> (element=w192:dbl[])  [unwired: 1 in]
                n141 = for {
                  tunnel: w190 -> [w195] mode=indexing
                  tunnel: w192 -> [w197]
                  tunnel: [w196] -> w187 mode=indexing
                  tunnel: w188 -> [w194] mode=indexing
                  n142 = Add(x=w195, y=w194) -> (x+y=w193:dbl[])
                  n143 = Subtract(x=w193, y=w197) -> (x-y=w196:dbl[])
                }
                n144 = property on="Lower chart" class="WFChart (strict)"("History Data"=w187) -> ()  [unwired: 2 in, 2 out]
              }
            }
          }
          event "Mixer freq [MHz]": Value Change {
            n145 = event-data() -> ()  [unwired: 1 in, 6 out]
            n146 = call-dynamic "SetMixerFrequency.vi"("Mixer freq [MHz]"="Mixer freq [MHz]", "Scope5785_six_channel"=w200) -> ("Scope5785_six_channel Out"=w198:refnum<class "Scope5782_six_channel.lvclass">)  [unwired: 8 in, 1 out]
          }
          event "Fequency [MHz]", "Phase offset (deg)": Value Change {
            n147 = event-data() -> ()  [unwired: 1 in, 6 out]
            n148 = call-dynamic "SetSimulatedFreq.vi"("Phase offset (deg)"="Phase offset (deg)", "Mixer freq [MHz]"="Fequency [MHz]", "Scope5785_six_channel"=w202) -> ("Scope5785_six_channel out"=w201:refnum<class "Scope5782_six_channel.lvclass">)  [unwired: 7 in, 1 out]
          }
          event "Output mixer fequency [MHz]", "Output enabled": Value Change {
            n149 = event-data() -> ()  [unwired: 1 in, 6 out]
            n150 = call "SetOutputFreq.vi"("Output enabled"="Output enabled", "Output mixer fequency [MHz]"="Output mixer fequency [MHz]", "Scope5785_six_channel"=w208) -> ("Scope5785_six_channel out"=w205:refnum<class "Scope5782_six_channel.lvclass">)  [unwired: 7 in, 1 out]
          }
          event "Output delay", "Output delay delta": Value Change {
            n151 = event-data() -> ()  [unwired: 1 in, 6 out]
            n152 = local read "Mixer freq [MHz]"() -> (w219:dbl)
            n153 = Multiply(x="Output delay", y=0.001) -> (x*y=w220:dbl)
            n154 = Multiply(x="Output delay delta", y=1e-06) -> (x*y=w222:dbl)
            n155 = Multiply(x=w219, y=6.283185307179586) -> (x*y=w217:dbl)
            n156 = Multiply(x=w217, y=w222) -> (x*y=w211:dbl)
            n157 = Multiply(x=w220, y=w217) -> (x*y=w214:dbl)
            n158 = call "Write Setting float.vi"("value"=w214, "FPGA Setting"=fpga_settings."Fi_start", "ScopeBase in"=w216) -> ("error out"=w212:errorcluster, "ScopeBase out"=w213:refnum<class "Scope5782_six_channel.lvclass">)  [unwired: 7 in]
            n159 = call "Write Setting float.vi"("error in (no error)"=w212, "value"=w211, "FPGA Setting"=fpga_settings."Fi_delta", "ScopeBase in"=w213) -> ("ScopeBase out"=w209:refnum<class "Scope5782_six_channel.lvclass">)  [unwired: 6 in, 1 out]
          }
          event "Fequency [kHz]", "a", "b": Value Change {
            n160 = event-data() -> ()  [unwired: 1 in, 6 out]
            n161 = call "SetAmPhase.vi"("b_am"="b", "a_am"="a", "fclk (MHz)"=100.0, "Am freq [kHz]"="Fequency [kHz]", "Scope5785_six_channel"=w231) -> ("Scope5785_six_channel out"=w230:refnum<class "Scope5782_six_channel.lvclass">)  [unwired: 5 in, 1 out]
          }
          event "Feedback", "Ki*T", "Kd/T", "Kp": Value Change {
            n162 = event-data() -> ()  [unwired: 1 in, 6 out]
            n163 = xnode "Reinterpret Number"("x"="Kd/T") -> ("y"=w249:fxp<+,32,32>)
            n164 = xnode "Reinterpret Number"("x"="Ki*T") -> ("y"=w248:fxp<+,32,32>)
            n165 = xnode "Reinterpret Number"("x"="Kp") -> ("y"=w250:fxp<+,32,32>)
            n166 = To Unsigned Long Integer(number=w248) -> (unsigned 32bit integer=w237:u32)
            n167 = To Unsigned Long Integer(number=w249) -> (unsigned 32bit integer=w236:u32)
            n168 = Boolean To (0,1)(Boolean="Feedback") -> (0, 1=w252:i16)
            n169 = To Unsigned Long Integer(number=w250) -> (unsigned 32bit integer=w235:u32)
            n170 = To Unsigned Long Integer(number=w252) -> (unsigned 32bit integer=w238:u32)
            n171 = call "Write Setting 32bit.vi"("value"=w238, "FPGA Setting"=fpga_settings."Feedback Enable", "ScopeBase in"=w244) -> ("ScopeBase out"=w243:refnum<class "Scope5782_six_channel.lvclass">)  [unwired: 7 in, 1 out]
            n172 = call "Write Setting 32bit.vi"("value"=w237, "FPGA Setting"=fpga_settings."Ki*Tau", "ScopeBase in"=w243) -> ("ScopeBase out"=w242:refnum<class "Scope5782_six_channel.lvclass">)  [unwired: 7 in, 1 out]
            n173 = call "Write Setting 32bit.vi"("value"=w236, "FPGA Setting"=fpga_settings."Kd_Tau", "ScopeBase in"=w242) -> ("ScopeBase out"=w241:refnum<class "Scope5782_six_channel.lvclass">)  [unwired: 7 in, 1 out]
            n174 = call "Write Setting 32bit.vi"("value"=w235, "FPGA Setting"=fpga_settings."Kp", "ScopeBase in"=w241) -> ("ScopeBase out"=w240:refnum<class "Scope5782_six_channel.lvclass">)  [unwired: 7 in, 1 out]
          }
          event "Feedback AM", "Ki*T AM", "Kd/T AM", "Kp AM": Value Change {
            n175 = event-data() -> ()  [unwired: 1 in, 6 out]
            n176 = xnode "Reinterpret Number"("x"="Kd/T AM") -> ("y"=w271:fxp<+,32,32>)
            n177 = xnode "Reinterpret Number"("x"="Ki*T AM") -> ("y"=w270:fxp<+,32,32>)
            n178 = xnode "Reinterpret Number"("x"="Kp AM") -> ("y"=w272:fxp<+,32,32>)
            n179 = To Unsigned Long Integer(number=w270) -> (unsigned 32bit integer=w255:u32)
            n180 = To Unsigned Long Integer(number=w271) -> (unsigned 32bit integer=w254:u32)
            n181 = Boolean To (0,1)(Boolean="Feedback AM") -> (0, 1=w273:i16)
            n182 = To Unsigned Long Integer(number=w272) -> (unsigned 32bit integer=w253:u32)
            n183 = To Unsigned Long Integer(number=w273) -> (unsigned 32bit integer=w259:u32)
            n184 = call "Write Setting 32bit.vi"("value"=w259, "FPGA Setting"=fpga_settings."Feedback AM", "ScopeBase in"=w262) -> ("ScopeBase out"=w265:refnum<class "Scope5782_six_channel.lvclass">)  [unwired: 7 in, 1 out]
            n185 = call "Write Setting 32bit.vi"("value"=w255, "FPGA Setting"=fpga_settings."Ki*Tau am", "ScopeBase in"=w265) -> ("ScopeBase out"=w264:refnum<class "Scope5782_six_channel.lvclass">)  [unwired: 7 in, 1 out]
            n186 = call "Write Setting 32bit.vi"("value"=w254, "FPGA Setting"=fpga_settings."Kd_Tau am", "ScopeBase in"=w264) -> ("ScopeBase out"=w263:refnum<class "Scope5782_six_channel.lvclass">)  [unwired: 7 in, 1 out]
            n187 = call "Write Setting 32bit.vi"("value"=w253, "FPGA Setting"=fpga_settings."Kp am", "ScopeBase in"=w263) -> ("ScopeBase out"=w261:refnum<class "Scope5782_six_channel.lvclass">)  [unwired: 7 in, 1 out]
          }
          event "w12", "R1", "w1", "Q1", "K1", "S": Value Change {
            n188 = event-data() -> ()  [unwired: 1 in, 6 out]
            n189 = call "CavityConstanstToFIFO.vi"("w12"="w12", "R1"="R1", "w1"="w1", "Q1"="Q1", "K1"="K1", "S"="S") -> ("FIFO array"=w276:u64[])  [unwired: 9 in]
            n190 = call "Write Setting Array.vi"("Data"=w276, "ScopeBase in"=w275) -> ("ScopeBase out"=w274:refnum<class "Scope5782_six_channel.lvclass">)  [unwired: 8 in, 1 out]
          }
          event "ch0 DC offset": Value Change {
            n191 = event-data() -> ()  [unwired: 1 in, 6 out]
            n192 = call "Read FpgaRef5782.vi"("Scope5785_six_channel"=w286) -> ("FpgaRef5782.lvclass"=w287:refnum<class "FpgaRef5782.lvclass">, "Scope5785_six_channel Out"=w285:refnum<class "Scope5782_six_channel.lvclass">)  [unwired: 8 in, 1 out]
            n193 = call "SetDcOffset.vi"("FPGA Setting"=fpga_settings."DC_offs 0", "DC offset"="ch0 DC offset", "FpgaRef5782 in"=w287) -> ()  [unwired: 7 in, 2 out]
          }
          event "ch0 DC offset 2": Value Change {
            n194 = event-data() -> ()  [unwired: 1 in, 6 out]
            n195 = call "Read FpgaRef5761.vi"("Scope5785_six_channel"=w291) -> ("FpgaRef5761.lvclass"=w292:refnum<class "FpgaRef5761.lvclass">, "Scope5785_six_channel Out"=w290:refnum<class "Scope5782_six_channel.lvclass">)  [unwired: 8 in, 1 out]
            n196 = call "SetDcOffset.vi"("FPGA Setting"=fpga_settings."DC_offs 0", "DC offset"="ch0 DC offset 2", "FpgaRef5761 In"=w292) -> ()  [unwired: 7 in, 2 out]
          }
          event "ch1 DC offset 2": Value Change {
            n197 = event-data() -> ()  [unwired: 1 in, 6 out]
            n198 = call "Read FpgaRef5761.vi"("Scope5785_six_channel"=w296) -> ("FpgaRef5761.lvclass"=w297:refnum<class "FpgaRef5761.lvclass">, "Scope5785_six_channel Out"=w295:refnum<class "Scope5782_six_channel.lvclass">)  [unwired: 8 in, 1 out]
            n199 = call "SetDcOffset.vi"("FPGA Setting"=fpga_settings."DC_offs 1", "DC offset"="ch1 DC offset 2", "FpgaRef5761 In"=w297) -> ()  [unwired: 7 in, 2 out]
          }
          event "ch2 DC offset": Value Change {
            n200 = event-data() -> ()  [unwired: 1 in, 6 out]
            n201 = call "Read FpgaRef5761.vi"("Scope5785_six_channel"=w301) -> ("FpgaRef5761.lvclass"=w302:refnum<class "FpgaRef5761.lvclass">, "Scope5785_six_channel Out"=w300:refnum<class "Scope5782_six_channel.lvclass">)  [unwired: 8 in, 1 out]
            n202 = call "SetDcOffset.vi"("FPGA Setting"=fpga_settings."DC_offs 2", "DC offset"="ch2 DC offset", "FpgaRef5761 In"=w302) -> ()  [unwired: 7 in, 2 out]
          }
          event "ch3 DC offset": Value Change {
            n203 = event-data() -> ()  [unwired: 1 in, 6 out]
            n204 = call "Read FpgaRef5761.vi"("Scope5785_six_channel"=w306) -> ("FpgaRef5761.lvclass"=w307:refnum<class "FpgaRef5761.lvclass">, "Scope5785_six_channel Out"=w305:refnum<class "Scope5782_six_channel.lvclass">)  [unwired: 8 in, 1 out]
            n205 = call "SetDcOffset.vi"("FPGA Setting"=fpga_settings."DC_offs 3", "DC offset"="ch3 DC offset", "FpgaRef5761 In"=w307) -> ()  [unwired: 7 in, 2 out]
          }
          event "Feedback delay", "Trigger delay": Value Change {
            n206 = event-data() -> ()  [unwired: 1 in, 6 out]
            n207 = Add(x="Feedback delay", y="Trigger delay") -> (x+y=w312:u32)
            n208 = call "Write Setting 32bit.vi"("value"=w312, "FPGA Setting"=fpga_settings."Feedback delay", "ScopeBase in"=w314) -> ("ScopeBase out"=w310:refnum<class "Scope5782_six_channel.lvclass">)  [unwired: 7 in, 1 out]
            n209 = call "Write Setting 32bit.vi"("value"="Trigger delay", "FPGA Setting"=fpga_settings."Trigger delay", "ScopeBase in"=w310) -> ("ScopeBase out"=w308:refnum<class "Scope5782_six_channel.lvclass">)  [unwired: 7 in, 1 out]
          }
          event "Acquire samples": Value Change {
            n210 = event-data() -> ()  [unwired: 1 in, 6 out]
            n211 = call "Write Setting 32bit.vi"("value"="Acquire samples", "FPGA Setting"=fpga_settings."Samples to acquire", "ScopeBase in"=w317) -> ("ScopeBase out"=w316:refnum<class "Scope5782_six_channel.lvclass">)  [unwired: 7 in, 1 out]
          }
          event "show setpoint": Value Change {
            n212 = event-data() -> ()  [unwired: 1 in, 6 out]
            n213 = call "Read Feedforward.vi"("Scope5785_six_channel"=w321) -> ("Feeforward"=w320:T20, "Scope5785_six_channel out"=w322:refnum<class "Scope5782_six_channel.lvclass">)  [unwired: 8 in, 1 out]
            n214 = Unbundle By Name(w320) -> ("Setpoint I"=w329:dbl[], "Setpoint Q"=w328:dbl[])
            n215 = Array Size(array=w329) -> (size(s)=w327:i32)
            n216 = Array Size(array=w328) -> (size(s)=w326:i32)
            n217 = Build Array(w329, w328) -> (w330:dbl[][])
            n218 = Greater Than 0?(x=w327) -> (x > 0?=w325:bool)
            n219 = Greater Than 0?(x=w326) -> (x > 0?=w324:bool)
            n220 = And(x=w325, y=w324) -> (x .and. y?=w323:bool)
            n221 = case shown="True" w323 {
              tunnel: w330 -> [_ w331]
              frame False {
              }
              frame True {
                n222 = call "ShowIQvaluesAsync.vi"("IQ data"=w331) -> ()  [unwired: 11 in]
              }
            }
          }
          event "show beam": Value Change {
            n223 = event-data() -> ()  [unwired: 1 in, 6 out]
            n224 = call "Read Feedforward.vi"("Scope5785_six_channel"=w334) -> ("Feeforward"=w332:T20, "Scope5785_six_channel out"=w333:refnum<class "Scope5782_six_channel.lvclass">)  [unwired: 8 in, 1 out]
            n225 = Unbundle By Name(w332) -> ("Beam I"=w341:dbl[], "Beam Q"=w340:dbl[])
            n226 = Array Size(array=w341) -> (size(s)=w339:i32)
            n227 = Array Size(array=w340) -> (size(s)=w338:i32)
            n228 = Build Array(w341, w340) -> (w342:dbl[][])
            n229 = Greater Than 0?(x=w339) -> (x > 0?=w337:bool)
            n230 = Greater Than 0?(x=w338) -> (x > 0?=w336:bool)
            n231 = And(x=w337, y=w336) -> (x .and. y?=w335:bool)
            n232 = case shown="True" w335 {
              tunnel: w342 -> [_ w343]
              frame False {
              }
              frame True {
                n233 = call "ShowIQvaluesAsync.vi"("IQ data"=w343) -> ()  [unwired: 11 in]
              }
            }
          }
          event "show feedforward": Value Change {
            n234 = event-data() -> ()  [unwired: 1 in, 6 out]
            n235 = call "Read Feedforward.vi"("Scope5785_six_channel"=w345) -> ("Feeforward"=w344:T20, "Scope5785_six_channel out"=w346:refnum<class "Scope5782_six_channel.lvclass">)  [unwired: 8 in, 1 out]
            n236 = Unbundle By Name(w344) -> ("Feedforward I"=w353:dbl[], "Feedforward Q"=w352:dbl[])
            n237 = Array Size(array=w353) -> (size(s)=w351:i32)
            n238 = Array Size(array=w352) -> (size(s)=w350:i32)
            n239 = Build Array(w353, w352) -> (w354:dbl[][])
            n240 = Greater Than 0?(x=w351) -> (x > 0?=w349:bool)
            n241 = Greater Than 0?(x=w350) -> (x > 0?=w348:bool)
            n242 = And(x=w349, y=w348) -> (x .and. y?=w347:bool)
            n243 = case shown="True" w347 {
              tunnel: w354 -> [_ w355]
              frame False {
              }
              frame True {
                n244 = call "ShowIQvaluesAsync.vi"("IQ data"=w355) -> ()  [unwired: 11 in]
              }
            }
          }
          event "ch1 DC offset": Value Change {
            n245 = event-data() -> ()  [unwired: 1 in, 6 out]
            n246 = call "Read FpgaRef5782.vi"("Scope5785_six_channel"=w360) -> ("FpgaRef5782.lvclass"=w357:refnum<class "FpgaRef5782.lvclass">, "Scope5785_six_channel Out"=w359:refnum<class "Scope5782_six_channel.lvclass">)  [unwired: 8 in, 1 out]
            n247 = call "SetDcOffset.vi"("FPGA Setting"=fpga_settings."DC_offs 1", "DC offset"="ch1 DC offset", "FpgaRef5782 in"=w357) -> ()  [unwired: 7 in, 2 out]
          }
          event "Setpoint enabled": Value Change {
            n248 = event-data() -> ()  [unwired: 1 in, 6 out]
            n249 = Boolean To (0,1)(Boolean="Setpoint enabled") -> (0, 1=w365:i16)
            n250 = To Word Integer(number=w365) -> (16bit integer=w367:i16)
            n251 = xnode "Reinterpret Number"("x"=w367) -> ("y"=w368:fxp<+/-,16,14>)
            n252 = xnode "Reinterpret Number"("x"=w368) -> ("y"=w364:fxp<+,16,16>)
            n253 = call "Write Setting 16bit.vi"("value"=w364, "FPGA Setting"=fpga_settings."Setpoint enable", "ScopeBase in"=w361) -> ("ScopeBase out"=w362:refnum<class "Scope5782_six_channel.lvclass">)  [unwired: 7 in, 1 out]
          }
          event "Beam/FF enabled": Value Change {
            n254 = event-data() -> ()  [unwired: 1 in, 6 out]
            n255 = Boolean To (0,1)(Boolean="Beam/FF enabled") -> (0, 1=w374:i16)
            n256 = To Word Integer(number=w374) -> (16bit integer=w375:i16)
            n257 = xnode "Reinterpret Number"("x"=w375) -> ("y"=w376:fxp<+/-,16,14>)
            n258 = xnode "Reinterpret Number"("x"=w376) -> ("y"=w371:fxp<+,16,16>)
            n259 = call "Write Setting 16bit.vi"("value"=w371, "FPGA Setting"=fpga_settings."Beam enable", "ScopeBase in"=w370) -> ("ScopeBase out"=w369:refnum<class "Scope5782_six_channel.lvclass">)  [unwired: 7 in, 1 out]
          }
          event "Cavity model": Value Change {
            n260 = event-data() -> ()  [unwired: 1 in, 6 out]
            n261 = Boolean To (0,1)(Boolean="Cavity model") -> (0, 1=w382:i16)
            n262 = To Word Integer(number=w382) -> (16bit integer=w383:i16)
            n263 = xnode "Reinterpret Number"("x"=w383) -> ("y"=w384:fxp<+/-,16,14>)
            n264 = xnode "Reinterpret Number"("x"=w384) -> ("y"=w377:fxp<+,16,16>)
            n265 = call "Write Setting 16bit.vi"("value"=w377, "FPGA Setting"=fpga_settings."Cavity Enable", "ScopeBase in"=w380) -> ("ScopeBase out"=w379:refnum<class "Scope5782_six_channel.lvclass">)  [unwired: 7 in, 1 out]
          }
          event Value Change {
            n266 = event-data() -> ()  [unwired: 1 in, 6 out]
            n267 = property on="Rumode" class="Bool (strict)"("Val(Sgnl)"=FALSE ("Value (Signaling)")) -> ()  [unwired: 2 in, 2 out]
            n268 = call-dynamic "SetMode.vi"("Mode"="Mode", "ScopeBase In"=w387) -> ("ScopeBase Out"=w385:refnum<class "Scope5782_six_channel.lvclass">)  [unwired: 8 in, 1 out]
          }
          event Value Change {
            n269 = event-data() -> ()  [unwired: 1 in, 6 out]
            n270 = call-dynamic "SetTrigger.vi"("Trigger"="Trigger", "ScopeBase In"=w391) -> ("ScopeBase Out"=w389:refnum<class "Scope5782_six_channel.lvclass">)  [unwired: 8 in, 1 out]
          }
          event "High speed transfer to host": Value Change {
            w398 = dbl[][] [] ("History Data")
            n271 = event-data() -> ()  [unwired: 1 in, 3 out]
            n272 = Multiply(x=10, y=w408) -> (x*y=w406:i32)
            n273 = Select(t=w406, s="High speed transfer to host", f=w408) -> (s? t:f=w394:i32)
            n274 = Select(t=0.0001, s="High speed transfer to host", f=0.001 ("t")) -> (s? t:f=w404:dbl)
            n275 = property on="Lower chart" class="WFChart (strict)"("History Data"=w398) -> ()  [unwired: 2 in, 2 out]
            n276 = property on="Upper chart" class="WFChart (strict)"("History Data"=w398) -> (error out=w399:errorcluster)  [unwired: 2 in, 1 out]
            n277 = Initialize Array(nan ("element"), 4 ("dimension size"), w394) -> (w401:dbl[][])
            n278 = property on="Upper chart" class="WFChart (strict)"("XScale.Multiplier"=w404) -> ()  [unwired: 2 in, 2 out]
            n279 = call-dynamic "SetRecordLength.vi"("Samples per 5782 record"=w394, "ScopeBase In"=w396) -> ("ScopeBase Out"=w395:refnum<class "Scope5782_six_channel.lvclass">)  [unwired: 8 in, 1 out]
            n280 = flat-sequence {
              tunnel: w401 -> [w410]
              tunnel: [w409] -> w397
              tunnel: w399 -> [_]
              frame #0 {
                n281 = local write "Upper chart"(w410) -> ()
                n282 = local read "Zoom time X"() -> (w409:bool)
              }
            }
            n283 = call-dynamic "SetFullSpeedTransfer.vi"("Full speed transfer"="High speed transfer to host", "ScopeBase In"=w395) -> ("ScopeBase Out"=w392:refnum<class "Scope5782_six_channel.lvclass">)  [unwired: 8 in, 1 out]
            n284 = property on="Zoom time X" class="Bool (strict)"("Val(Sgnl)"=w397) -> ()  [unwired: 2 in, 2 out]
          }
          event "Samples per 5782 record": Value Change {
            n285 = event-data() -> ()  [unwired: 1 in, 6 out]
            n286 = call-dynamic "SetRecordLength.vi"("Samples per 5782 record"="Samples per 5782 record", "ScopeBase In"=w413) -> ("ScopeBase Out"=w411:refnum<class "Scope5782_six_channel.lvclass">)  [unwired: 8 in, 1 out]
          }
          event "Singleshot": Value Change {
            n287 = event-data() -> ()  [unwired: 1 in, 6 out]
            n288 = local write "Rumode"(FALSE ("Rumode")) -> ()
            n289 = call-dynamic "SetRunMode.vi"("RunMode"=ScopeMode."Single" ("scope mode"), "ScopeBase in"=w414) -> ("ScopeBase out"=w415:refnum<class "Scope5782_six_channel.lvclass">)  [unwired: 8 in, 1 out]
          }
          event "Rumode": Value Change {
            n290 = event-data() -> ()  [unwired: 1 in, 6 out]
            n291 = case shown="\"Triggered\"" "Trigmode" {
              tunnel: [ScopeMode."Running" ("scope mode") ScopeMode."Continuous" ("scope mode")] -> w421
              frame "Triggered" {
              }
              frame "Continuous" {
              }
            }
            n292 = Select(t=w421, s="Rumode", f=ScopeMode."Stopped" ("scope mode")) -> (s? t:f=w420:T19)
            n293 = call-dynamic "SetRunMode.vi"("RunMode"=w420, "ScopeBase in"=w419) -> ("ScopeBase out"=w418:refnum<class "Scope5782_six_channel.lvclass">)  [unwired: 8 in, 1 out]
          }
          event "unwrap phase": Value Change {
            w427 = dbl[][] [] ("History Data")
            n294 = event-data() -> ()  [unwired: 1 in, 6 out]
            n295 = property on="Lower chart" class="WFChart (strict)"("History Data"=w427) -> ()  [unwired: 2 in, 2 out]
            n296 = property on="Upper chart" class="WFChart (strict)"("History Data"=w427) -> ()  [unwired: 2 in, 2 out]
          }
          event "stop": Value Change {
            n297 = event-data() -> ()  [unwired: 1 in, 6 out]
          }
          event Value Change {
            n298 = event-data() -> ()  [unwired: 1 in, 6 out]
            n299 = case shown="\"V\"" "Unit" {
              tunnel: ["V" "dBV" "V^2"] -> w433
              frame "V" {
              }
              frame "dBV" {
              }
              frame "V^2" {
              }
            }
            n300 = Concatenate Strings("Amplitude [", w433, "]") -> (w431:string)
            n301 = property on="freqdata" class="WFGraph (strict)"("YScale.NameLbl.Text"=w431) -> ()  [unwired: 2 in, 2 out]
          }
          event "#bins": Value Change {
            n302 = event-data() -> ()  [unwired: 1 in, 6 out]
            n303 = local read "Upper chart"() -> (w443:dbl[][])
            n304 = local read "Window"() -> (w444:T6)
            n305 = local read "Unit"() -> (w445:T5)
            n306 = call "calc FFT_indexed.vi"("#bins"="#bins", "IQ indexes"=i32[][] [[0, 1], [2, 3], [4, 5], [6, 7], [8, 9], [10, 11], [12, 13]], "dt"=1e-06, "Unit"=w445, "Window"=w444, "data"=w443) -> ("Power Spectrum / PSD"=w442:cluster{"f0":dbl, "df":dbl, "magnitude":dbl[]}[])  [unwired: 5 in]
            n307 = local write "freqdata"(w442) -> ()
          }
          event "Zoom time X", "Zoom time Y": Value Change {
            n308 = event-data() -> ()  [unwired: 1 in, 6 out]
            n309 = control-ref of="Upper chart"() -> (w450:refnum<vi>)
            n310 = control-ref of="Upper graph"() -> (w451:refnum<vi>)
            n311 = call "setZoomTool.vi"("Zoom Y"="Zoom time Y", "Zoom  X"="Zoom time X", "reference"=w450) -> ()  [unwired: 9 in]
            n312 = call "setZoomTool.vi"("Zoom Y"="Zoom time Y", "Zoom  X"="Zoom time X", "reference"=w451) -> ()  [unwired: 9 in]
          }
          event "Zoom freq Y", "Zoom freq X": Value Change {
            n313 = event-data() -> ()  [unwired: 1 in, 6 out]
            n314 = control-ref of="Lower chart"() -> (w456:refnum<vi>)
            n315 = control-ref of="Lower graph"() -> (w455:refnum<vi>)
            n316 = control-ref of="freqdata"() -> (w457:refnum<vi>)
            n317 = call "setZoomTool.vi"("Zoom Y"="Zoom freq Y", "Zoom  X"="Zoom freq X", "reference"=w457) -> ()  [unwired: 9 in]
            n318 = call "setZoomTool.vi"("Zoom Y"="Zoom freq Y", "Zoom  X"="Zoom freq X", "reference"=w456) -> ()  [unwired: 9 in]
            n319 = call "setZoomTool.vi"("Zoom Y"="Zoom freq Y", "Zoom  X"="Zoom freq X", "reference"=w455) -> ()  [unwired: 9 in]
          }
          event Value Change {
            w461 = dbl[][] [] ("History Data")
            n320 = event-data() -> ()  [unwired: 1 in, 6 out]
            n321 = property on="Upper chart" class="WFChart (strict)"("History Data"=w461) -> ()  [unwired: 2 in, 2 out]
            n322 = property on="Lower chart" class="WFChart (strict)"("History Data"=w461) -> ()  [unwired: 2 in, 2 out]
            n323 = local write "freqdata"(cluster{"f0":dbl, "df":dbl, "magnitude":dbl[]}[] [] ("freqdata")) -> ()
            n324 = call "UpdateGraphs.vi"("Buffer mode"="Buffer", "Display mode"="Display", "Graph_refs"=w462) -> ()  [unwired: 9 in]
            n325 = property on="Zoom time X" class="Bool (strict)"("Val(Sgnl)"=TRUE ("Value (Signaling)")) -> ()  [unwired: 2 in, 2 out]
          }
          event "Feed forward": Value Change {
            n326 = event-data() -> ()  [unwired: 1 in, 6 out]
            n327 = control-ref of="show feedforward"() -> (w472:refnum<vi>)
            n328 = call "LoadFeedforward.vi"("show ref"=w472, "Path"="Feed forward") -> ("error out"=w467:errorcluster, "values Q"=w468:dbl[], "values I"=w469:dbl[])  [unwired: 7 in]
            n329 = call "SetFeedForward.vi"("error in (no error)"=w467, "values Q"=w468, "values I"=w469, "Scope5785_six_channel"=w470) -> ("Scope5785_six_channel out"=w466:refnum<class "Scope5782_six_channel.lvclass">)  [unwired: 6 in, 1 out]
          }
          event "Beam": Value Change {
            n330 = event-data() -> ()  [unwired: 1 in, 6 out]
            n331 = control-ref of="show beam"() -> (w479:refnum<vi>)
            n332 = call "LoadFeedforward.vi"("show ref"=w479, "Path"="Beam") -> ("error out"=w473:errorcluster, "values Q"=w476:dbl[], "values I"=w477:dbl[])  [unwired: 7 in]
            n333 = call "SetBeam.vi"("error in (no error)"=w473, "values Q"=w476, "values I"=w477, "Scope5785_six_channel"=w475) -> ("Scope5785_six_channel out"=w474:refnum<class "Scope5782_six_channel.lvclass">)  [unwired: 6 in, 1 out]
          }
          event "Setpoint": Value Change {
            n334 = event-data() -> ()  [unwired: 1 in, 6 out]
            n335 = control-ref of="show setpoint"() -> (w486:refnum<vi>)
            n336 = call "LoadFeedforward.vi"("show ref"=w486, "Path"="Setpoint") -> ("error out"=w481:errorcluster, "values Q"=w483:dbl[], "values I"=w484:dbl[])  [unwired: 7 in]
            n337 = call "SetSetpoint.vi"("error in (no error)"=w481, "values Q"=w483, "values I"=w484, "Scope5785_six_channel"=w482) -> ("Scope5785_six_channel out"=w480:refnum<class "Scope5782_six_channel.lvclass">)  [unwired: 6 in, 1 out]
          }
          event "Input delay 5782": Value Change {
            n338 = event-data() -> ()  [unwired: 1 in, 6 out]
            n339 = call "Read FpgaRef5782.vi"("Scope5785_six_channel"=w491) -> ("FpgaRef5782.lvclass"=w490:refnum<class "FpgaRef5782.lvclass">, "Scope5785_six_channel Out"=w487:refnum<class "Scope5782_six_channel.lvclass">)  [unwired: 8 in, 1 out]
            n340 = call "WriteSetting 32bit.vi"("value"="Input delay 5782", "FPGA Setting"=fpga_settings."Input delay", "FpgaRefBase in"=w490) -> ()  [unwired: 7 in, 2 out]
          }
          event "Input delay 5761": Value Change {
            n341 = event-data() -> ()  [unwired: 1 in, 6 out]
            n342 = call "Read FpgaRef5761.vi"("Scope5785_six_channel"=w496) -> ("FpgaRef5761.lvclass"=w495:refnum<class "FpgaRef5761.lvclass">, "Scope5785_six_channel Out"=w493:refnum<class "Scope5782_six_channel.lvclass">)  [unwired: 8 in, 1 out]
            n343 = call "WriteSetting 32bit.vi"("value"="Input delay 5761", "FPGA Setting"=fpga_settings."Input delay", "FpgaRefBase in"=w495) -> ()  [unwired: 7 in, 2 out]
          }
        }
      }
      "stop 2" <- w112
    }
    frame Error {
    }
  }
  n344 = Unregister For Events(event registration refnum=w77) -> ()  [unwired: 1 in, 1 out]
  n345 = call-dynamic "Close.vi"("ScopeBase in"=w23) -> ("error out"=w22:errorcluster)  [unwired: 10 in]
  n346 = flat-sequence {
    tunnel: w22 -> [_]
    frame #0 {
      n347 = global write "global_stop.vi" "Stop"(TRUE ("Stop")) -> ()
    }
  }
